vi "move_to_position (SubVI).vi"(9 "error in (no error)":errorcluster, 10 "Cluster":cluster{dbl, dbl, dbl}, 11 ".NET Refnum in":refnum<k24>) -> (0 "Current Z":dbl, 1 "error out":errorcluster, 3 ".NET Refnum out":refnum<k24>, 4 "Current Y":dbl, 6 "Current X":dbl)   [LabVIEW 2026]
uses:
  C:/Program Files (x86)/Control/SC3U.dll
  Program Files (x86)/Control/SC3U.dll
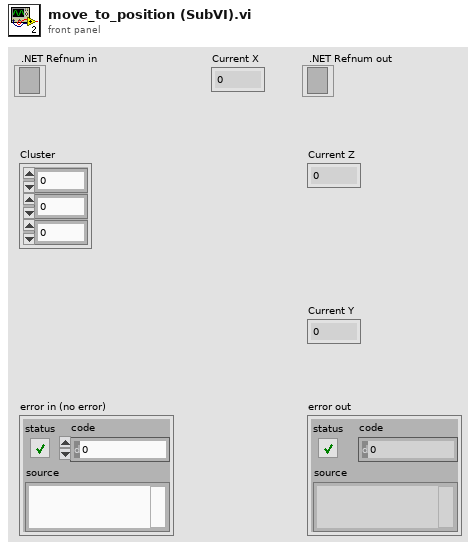
[diagram p1: front panel]
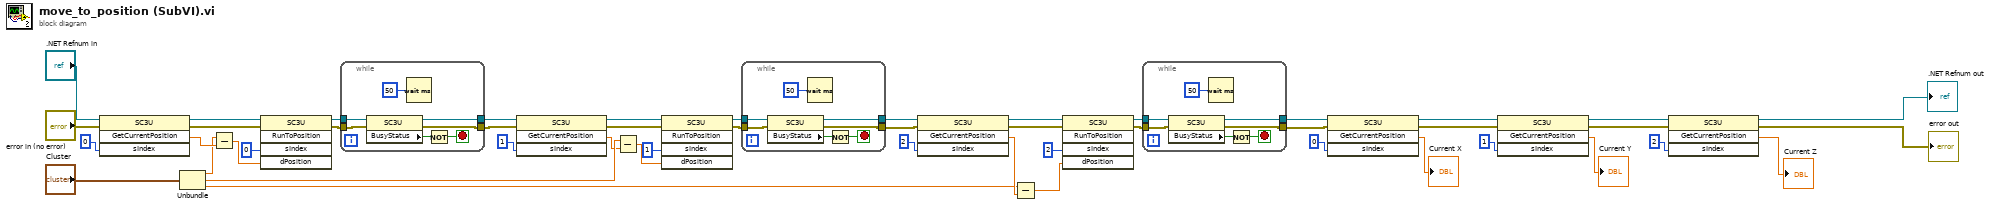
[diagram p0: block diagram]
diagram:
  n1 = invoke class="SC3U" method="GetCurrentPosition"(reference=".NET Refnum in", error in="error in (no error)", "sIndex"=i16 0) -> (reference out=w33:refnum<k24>, error out=w48:errorcluster, "GetCurrentPosition"=w31:dbl)  [unwired: 1 in, 1 out]
  n2 = Unbundle("Cluster") -> (w30:dbl, w28:dbl, w24:dbl)
  n3 = Subtract(x=w30, y=w31) -> (x-y=w32:dbl)
  n4 = invoke class="SC3U" method="RunToPosition"(reference=w33, error in=w48, "sIndex"=i16 0, "dPosition"=w32) -> (reference out=w5:refnum<k24>, error out=w47:errorcluster)  [unwired: 1 in, 3 out]
  n5 = while {
    tunnel: w5 -> [w52]
    tunnel: [w51] -> w18
    tunnel: [w50] -> w46
    tunnel: w47 -> [w49]
    stop <- w54 stop-if-true
    n6 = property class="SC3U"(reference=w52, error in=w49) -> (reference out=w51:refnum<k24>, error out=w50:errorcluster, "BusyStatus"=w53:bool)
    n7 = Wait (ms)(milliseconds to wait=u32 50) -> ()  [unwired: 1 out]
    n8 = Not(x=w53) -> (.not. x?=w54:bool)
  }
  n9 = invoke class="SC3U" method="GetCurrentPosition"(reference=w18, error in=w46, "sIndex"=i16 1) -> (reference out=w19:refnum<k24>, error out=w45:errorcluster, "GetCurrentPosition"=w27:dbl)  [unwired: 1 in, 1 out]
  n10 = Subtract(x=w28, y=w27) -> (x-y=w29:dbl)
  n11 = invoke class="SC3U" method="RunToPosition"(reference=w19, error in=w45, "sIndex"=i16 1, "dPosition"=w29) -> (reference out=w20:refnum<k24>, error out=w44:errorcluster)  [unwired: 1 in, 3 out]
  n12 = while {
    tunnel: w20 -> [w59]
    tunnel: [w58] -> w15
    tunnel: [w57] -> w43
    tunnel: w44 -> [w56]
    stop <- w61 stop-if-true
    n13 = property class="SC3U"(reference=w59, error in=w56) -> (reference out=w58:refnum<k24>, error out=w57:errorcluster, "BusyStatus"=w60:bool)
    n14 = Wait (ms)(milliseconds to wait=u32 50) -> ()  [unwired: 1 out]
    n15 = Not(x=w60) -> (.not. x?=w61:bool)
  }
  n16 = invoke class="SC3U" method="GetCurrentPosition"(reference=w15, error in=w43, "sIndex"=i16 2) -> (reference out=w16:refnum<k24>, error out=w42:errorcluster, "GetCurrentPosition"=w25:dbl)  [unwired: 1 in, 1 out]
  n17 = Subtract(x=w24, y=w25) -> (x-y=w26:dbl)
  n18 = invoke class="SC3U" method="RunToPosition"(reference=w16, error in=w42, "sIndex"=i16 2, "dPosition"=w26) -> (reference out=w17:refnum<k24>, error out=w41:errorcluster)  [unwired: 1 in, 3 out]
  n19 = while {
    tunnel: w17 -> [w66]
    tunnel: [w65] -> w7
    tunnel: [w64] -> w40
    tunnel: w41 -> [w63]
    stop <- w68 stop-if-true
    n20 = property class="SC3U"(reference=w66, error in=w63) -> (reference out=w65:refnum<k24>, error out=w64:errorcluster, "BusyStatus"=w67:bool)
    n21 = Wait (ms)(milliseconds to wait=u32 50) -> ()  [unwired: 1 out]
    n22 = Not(x=w67) -> (.not. x?=w68:bool)
  }
  n23 = invoke class="SC3U" method="GetCurrentPosition"(reference=w7, error in=w40, "sIndex"=i16 0 ("iAxis")) -> (reference out=w10:refnum<k24>, error out=w39:errorcluster, "GetCurrentPosition"=→"Current X":dbl)  [unwired: 1 in, 1 out]
  n24 = invoke class="SC3U" method="GetCurrentPosition"(reference=w10, error in=w39, "sIndex"=i16 1 ("iAxis")) -> (reference out=w11:refnum<k24>, error out=w38:errorcluster, "GetCurrentPosition"=→"Current Y":dbl)  [unwired: 1 in, 1 out]
  n25 = invoke class="SC3U" method="GetCurrentPosition"(reference=w11, error in=w38, "sIndex"=i16 2 ("iAxis")) -> (reference out=→".NET Refnum out":refnum<k24>, error out=→"error out":errorcluster, "GetCurrentPosition"=→"Current Z":dbl)  [unwired: 1 in, 1 out]
